vi "Utility Get Build Version.vi"(7 "VI Ref in":refnum<vi>, 9 "Version Index (2:Fix, +1:Build)":i32=2, 10 "Name of build specification":string) -> (1 "Rev (Build)":u16, 2 "Version (Fix)":u16, 4 "error out":errorcluster)   [LabVIEW 2015]
uses:
  <vilib>/AppBuilder/AB_API_Simple/Build Specification Version.ctl
  <vilib>/AppBuilder/AB_API_Simple/Get Build Specification Version (path).vi
  <vilib>/AppBuilder/AB_API_Simple/NI_App_Builder_API.lvlib
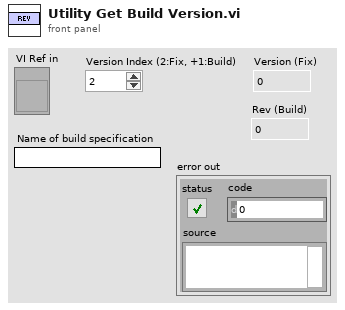
[diagram p1: front panel]
types:
  T1 = typedef "NI_App_Builder_API.lvlib/Build Specification Version.ctl" = cluster{"Major":u16, "Minor":u16, "Fix":u16, "Build":u16}
  T2 = cluster{"last mod":timestamp, "appended path":path}
  T3 = cluster{"last mod":timestamp, "appended path":path}[]
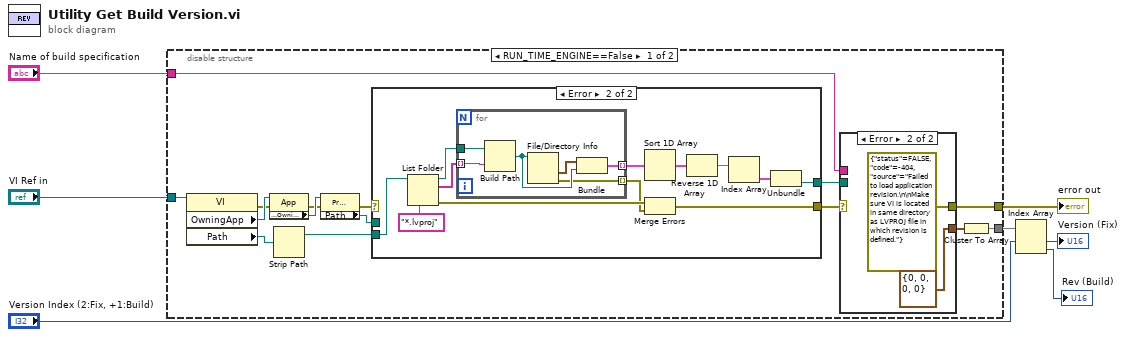
[diagram p0: block diagram]
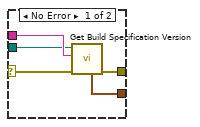
[diagram p3: hidden frame]
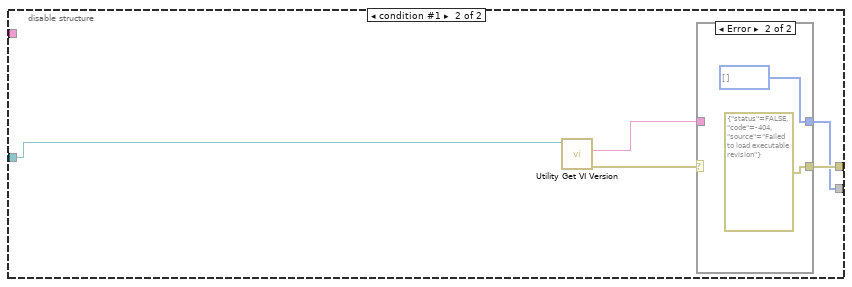
[diagram p4: hidden frame]
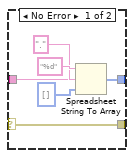
[diagram p5: hidden frame]
diagram:
  n1 = disable-structure shown="RUN_TIME_ENGINE==False" {
    disable-tunnel: [w17 w51] -> w4
    disable-tunnel: "VI Ref in" -> [w22 w54]
    disable-tunnel: "Name of build specification" -> [w19 _]
    disable-tunnel: [w14 w52] -> w2
    frame condition #0 (active) {
      n2 = property class="VI"(reference=w22) -> (error out=w15:errorcluster, "OwningApp"=w21:refnum<vi>, "Path"=w10:path)  [unwired: 1 in, 1 out]
      n3 = property class="App"(reference=w21, error in=w15) -> (error out=w16:errorcluster, "Project.OwningProject"=w20:refnum<vi>)  [unwired: 1 out]
      n4 = Strip Path(path=w10) -> (stripped path=w9:path)  [unwired: 1 out]
      n5 = property class="Project"(reference=w20, error in=w16) -> (error out=w11:errorcluster, "Path"=w12:path)  [unwired: 1 out]
      n6 = case shown="Error" w11 {
        selector: w11 -> [w23 _]
        tunnel: [w24 w28] -> w13
        tunnel: w12 -> [w24 _]
        tunnel: w9 -> [_ w34]
        tunnel: [w23 w25] -> w8
        frame No Error {
        }
        frame Error {
          n7 = List Folder(path=w34, pattern="*.lvproj") -> (path out=w33:path, filenames=w32:string[], error out=w27:errorcluster)  [unwired: 2 in, 1 out]
          n8 = for {
            tunnel: w33 -> [w42]
            tunnel: w32 -> [w41] mode=indexing
            tunnel: [w38] -> w36 mode=indexing
            tunnel: [w37] -> w26 mode=indexing
            n9 = Build Path(base path=w42, name or relative path=w41) -> (appended path=w39:path)
            n10 = File/Directory Info(path=w39) -> (last mod=w40:timestamp, error out=w37:errorcluster)  [unwired: 1 in, 5 out]
            n11 = Bundle("last mod"=w40, "appended path"=w39) -> (w38:T2)  [unwired: 1 in]
          }
          n12 = Sort 1D Array(array=w36) -> (sorted array=w31:T3)
          n13 = Merge Errors(w27, w26) -> (w25:errorcluster)
          n14 = Reverse 1D Array(array=w31) -> (reversed array=w30:T3)
          n15 = Index Array(array=w30) -> (element=w29:T2)  [unwired: 1 in]
          n16 = Unbundle(w29) -> ("appended path"=w28:path)  [unwired: 1 out]
        }
      }
      n17 = case shown="Error" w8 {
        selector: w8 -> [w43 _]
        tunnel: w19 -> [w47 _]
        tunnel: [w46 T1 {"Major"=0, "Minor"=0, "Fix"=0, "Build"=0} ("Build Specification Version")] -> w18
        tunnel: [w45 errorcluster {"status"=FALSE, "code"=-404, "source"="Failed to load application revision.\n\nMake sure VI is located in same directory as LVPROJ file in which revision is defined."} ("error out")] -> w14
        tunnel: w13 -> [w44 _]
        frame No Error {
          n18 = call-poly <vilib>:"Get Build Specification Version.vi"("error in (no error)"=w43, "Name of build specification"=w47, "Path to project"=w44) -> ("error out"=w45:errorcluster, "Build Specification Version"=w46:T1)  [unwired: 7 in]
        }
        frame Error {
        }
      }
      n19 = Cluster To Array(cluster=w18) -> (array=w17:u16[])
    }
    frame condition #1 {
      n20 = call "Utility Get VI Version.vi"("VI in"=w54) -> ("error out"=w53:errorcluster, "version"=w50:string)  [unwired: 8 in, 1 out]
      n21 = case shown="Error" w53 {
        selector: w53 -> [w60 _]
        tunnel: [w60 errorcluster {"status"=FALSE, "code"=-404, "source"="Failed to load executable revision"} ("error out")] -> w52
        tunnel: w50 -> [w56 _]
        tunnel: [w55 u16[] []] -> w51
        frame No Error {
          n22 = Spreadsheet String To Array(delimiter (Tab)=".", format string="%d", spreadsheet string=w56, array type (2D Dbl)=u16[] []) -> (array=w55:u16[])
        }
        frame Error {
        }
      }
    }
  }
  "error out" <- w2
  n23 = Index Array(array=w4, index #1="Version Index (2:Fix, +1:Build)") -> (element #1=→"Version (Fix)":u16, element #2=→"Rev (Build)":u16)  [unwired: 1 in]
